vi "Stabilize.vi"() -> ()   [LabVIEW 2013]
uses:
  <vilib>/vision/NI_Vision_Development_Module.lvlib
panel:
  in  "Frame for Template":u32=5000
  out "Match Quality":sgl(graph)
  in  "Stop Updating Panel":bool
  out "Total # Of Frames:":dbl
  out "Stabilized":T1(plugin-control)
  out "Original":T1(plugin-control)
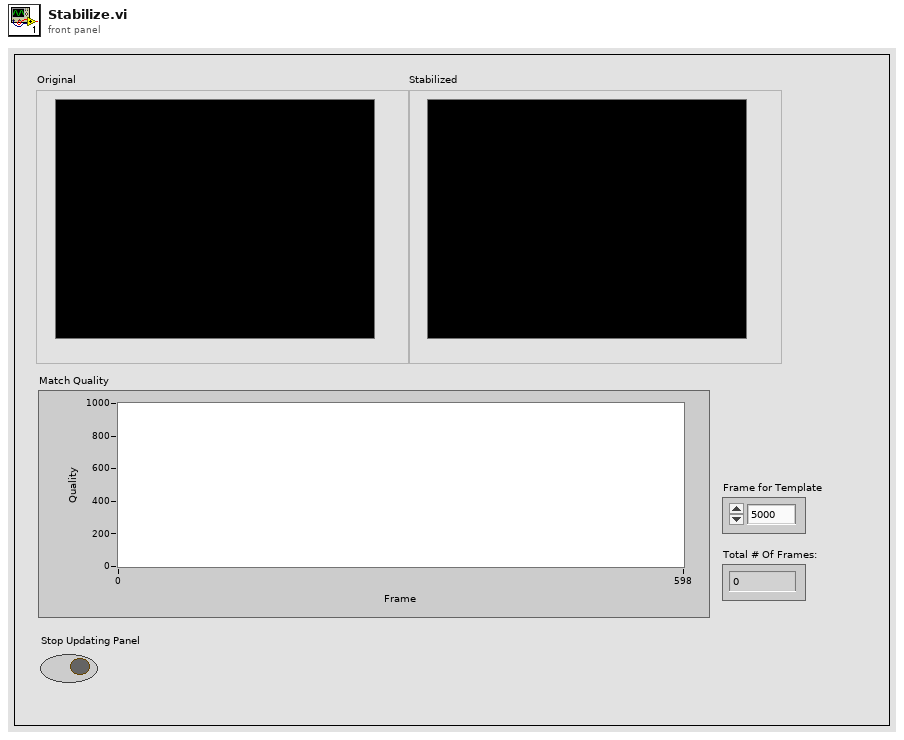
[diagram p1: front panel]
types:
  T1 = typedef "IMAQ Image.ctl" = refnum<image>
  T2 = typedef "AviRefnum.ctl" = refnum<k1>
  T3 = cluster{"width":u32, "height":u32, "framesPerSecond":u32, "compressionFilter":string, "hasData":bool}
  T4 = typedef "IMAQ Rectangle" = cluster{"Left":i32, "Top":i32, "Right":i32, "Bottom":i32, "Rotation":dbl}
  T5 = typedef "ROI Descriptor" = cluster{"Global Rectangle":i32[], "Contours":cluster{"ID":enum32{"External", "Internal"}, "Type":u32, "Coordinates":i32[]}[]}
  T6 = cluster{"Position":cluster{"x":sgl, "y":sgl}, "Angle":sgl, "Scale":sgl, "Score":sgl, "Bounding Box":cluster{"x":sgl, "y":sgl}[]}[]
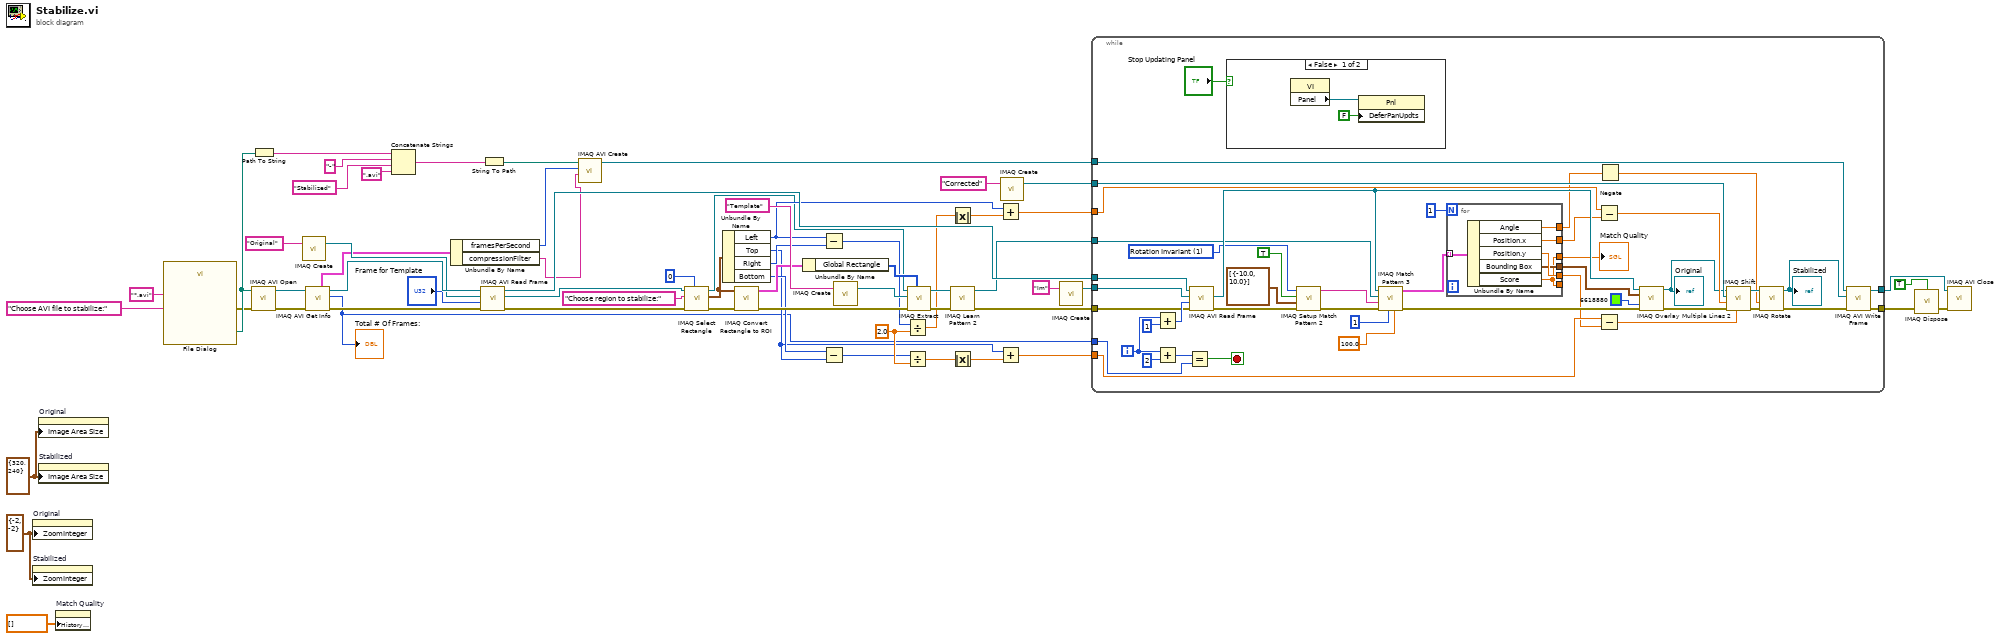
[diagram p0: block diagram]
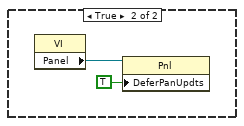
[diagram p2: hidden frame]
diagram:
  w22 = cluster{"X":i32, "Y":i32} {"X"=-2, "Y"=-2} ("ZoomInteger:All Elements")
  w23 = cluster{"Width":u32, "Height":u32} {"Width"=320, "Height"=240} ("Image Area:Size:All Elements")
  w47 = 2.0 ("y")
  n1 = property on="Original" class="ImageControl"("ZoomInteger"=w22) -> ()  [unwired: 2 in, 2 out]
  n2 = property on="Stabilized" class="ImageControl"("ZoomInteger"=w22) -> ()  [unwired: 2 in, 2 out]
  n3 = property on="Original" class="ImageControl"("Image Area Size"=w23) -> ()  [unwired: 2 in, 2 out]
  n4 = property on="Stabilized" class="ImageControl"("Image Area Size"=w23) -> ()  [unwired: 2 in, 2 out]
  n5 = property on="Match Quality" class="WFChart (strict)"("History Data"=sgl[] []) -> ()  [unwired: 2 in, 2 out]
  n6 = call "File Dialog"("prompt"="Choose AVI file to stabilize:", "pattern label"="*.avi") -> ("selected path"=w5:path, "error out"=w3:errorcluster)  [unwired: 10 in, 2 out]
  n7 = call "IMAQ AVI Open"("error in (no error)"=w3, "AVI Path"=w5) -> ("error out"=w62:errorcluster, "Avi Refnum"=w63:T2)  [unwired: 8 in]
  n8 = Path To String(path=w5) -> (string=w10:string)
  n9 = call "IMAQ Create"("Image Name"="Original") -> ("New Image"=w59:T1)  [unwired: 4 in, 1 out]
  n10 = call "IMAQ AVI Get Info"("error in (no error)"=w62, "Avi Refnum"=w63) -> ("error out"=w58:errorcluster, "Number of Frames"=w19:u32, "Avi Refnum (duplicate)"=w61:T2, "Frame Data"=w38:T3)  [unwired: 5 in, 1 out]
  "Total # Of Frames:" <- w19
  n11 = Concatenate Strings(w10, "-" ("string"), "Stabilized" ("string"), ".avi" ("string")) -> (w7:string)
  n12 = Unbundle By Name(w38) -> ("framesPerSecond"=w37:u32, "compressionFilter"=w1:string)
  n13 = call "IMAQ AVI Read Frame"("error in (no error)"=w58, "Frame Number"="Frame for Template", "Image"=w59, "Avi Refnum"=w61) -> ("error out"=w25:errorcluster, "Image Out"=w57:T1, "Avi Refnum (duplicate)"=w48:T2)  [unwired: 4 in, 1 out]
  n14 = String To Path(string=w7) -> (path=w4:path)
  n15 = call "IMAQ AVI Create"("Compression Filter"=w1, "Frames Per Second"=w37, "AVI Path"=w4) -> ("Avi Refnum"=w36:T2)  [unwired: 7 in, 1 out]
  n16 = call "IMAQ Select Rectangle"("Window Number (0...15)"=0, "error in (no error)"=w25, "Prompt"="Choose region to stabilize:", "Image In"=w57) -> ("error out"=w27:errorcluster, "Rectangle"=w18:T4, "Image Out (duplicate)"=w30:T1)  [unwired: 4 in, 1 out]
  n17 = Unbundle By Name(w18) -> ("Left"=w42:i32, "Top"=w41:i32, "Right"=w44:i32, "Bottom"=w43:i32)
  n18 = call "IMAQ Convert Rectangle to ROI"("error in (no error)"=w27, "Rectangle"=w18) -> ("error out"=w53:errorcluster, "ROI Descriptor"=w52:T5)  [unwired: 7 in]
  n19 = Unbundle By Name(w52) -> ("Global Rectangle"=w51:i32[])
  n20 = Subtract(x=w42, y=w44) -> (x-y=w46:i32)
  n21 = Subtract(x=w43, y=w41) -> (x-y=w45:i32)
  n22 = call "IMAQ Create"("Image Name"="Template") -> ("New Image"=w54:T1)  [unwired: 4 in, 1 out]
  n23 = Divide(x=w46, y=w47) -> (x/y=w35:dbl)
  n24 = Divide(x=w45, y=w47) -> (x/y=w33:dbl)
  n25 = call "IMAQ Extract"("Optional Rectangle"=w51, "error in (no error)"=w53, "Image Dst"=w54, "Image Src"=w30) -> ("error out"=w49:errorcluster, "Image Dst Out"=w50:T1)  [unwired: 6 in]
  n26 = Absolute Value(x=w35) -> (abs(x)=w34:dbl)
  n27 = call "IMAQ Learn Pattern 2"("error in (no error)"=w49, "Image"=w50) -> ("error out"=w24:errorcluster, "Template Image Out"=w31:T1)  [unwired: 8 in]
  n28 = Absolute Value(x=w33) -> (abs(x)=w32:dbl)
  n29 = Add(x=w42, y=w34) -> (x+y=w40:dbl)
  n30 = Add(x=w41, y=w32) -> (x+y=w39:dbl)
  n31 = call "IMAQ Create"("Image Name"="Corrected") -> ("New Image"=w14:T1)  [unwired: 4 in, 1 out]
  n32 = call "IMAQ Create"("Image Name"="Im") -> ("New Image"=w16:T1)  [unwired: 4 in, 1 out]
  n33 = while {
    tunnel: w48 -> [w108]
    tunnel: w19 -> [w102]
    tunnel: w31 -> [w87]
    tunnel: w40 -> [w98]
    tunnel: w39 -> [w96]
    tunnel: w36 -> [w94]
    tunnel: w24 -> [w81]
    tunnel: [w84] -> w21
    tunnel: w16 -> [w82]
    tunnel: w14 -> [w79]
    tunnel: [w78] -> w12
    i -> [w105]
    stop <- w101 stop-if-true
    w71 = u16 1 items=["Shift Invariant", "Rotation Invariant"] ("Match Mode")
    n34 = Add(x=w105, y=1) -> (x+y=w106:i32)
    n35 = Add(x=w105, y=2) -> (x+y=w103:i32)
    n36 = Equal?(x=w103, y=w102) -> (x = y?=w101:bool)
    n37 = call "IMAQ AVI Read Frame"("error in (no error)"=w81, "Frame Number"=w106, "Image"=w82, "Avi Refnum"=w108) -> ("error out"=w90:errorcluster, "Image Out"=w92:T1)  [unwired: 4 in, 2 out]
    n38 = case shown="False" "Stop Updating Panel" {
      frame False {
        n39 = property class="VI"() -> ("Panel"=w109:refnum<vi>)  [unwired: 2 in, 2 out]
        n40 = property class="Pnl"(reference=w109, "DeferPanUpdts"=FALSE ("Defer Panel Updates")) -> ()  [unwired: 1 in, 2 out]
      }
      frame True {
        n41 = property class="VI"() -> ("Panel"=w111:refnum<vi>)  [unwired: 2 in, 2 out]
        n42 = property class="Pnl"(reference=w111, "DeferPanUpdts"=TRUE ("Defer Panel Updates")) -> ()  [unwired: 1 in, 2 out]
      }
    }
    n43 = call "IMAQ Setup Match Pattern 2"("error in (no error)"=w90, "Rotation Angle Ranges (degrees)"=cluster{sgl, sgl}[] [{-10.0, 10.0}], "Subpixel Accuracy"=TRUE, "Match Mode"=w71) -> ("error out"=w89:errorcluster, "Match Pattern Setup Data"=w88:string)  [unwired: 6 in]
    n44 = call "IMAQ Match Pattern 3"("Minimum Match Score"=sgl 100.0, "Number of Matches Requested"=1, "error in (no error)"=w89, "Match Pattern Setup Data"=w88, "Template Image"=w87, "Image"=w92) -> ("error out"=w80:errorcluster, "Matches"=w100:T6)  [unwired: 3 in, 1 out]
    n45 = for {
      N: 1 -> [_]
      tunnel: w100 -> [w118] mode=indexing
      tunnel: [w117] -> w77
      tunnel: [w116] -> w76
      tunnel: [w115] -> w93
      tunnel: [w114] -> w85
      tunnel: [w114] -> _
      tunnel: [w113] -> w68
      n46 = Unbundle By Name(w118) -> ("Angle"=w113:sgl, "Position.x"=w117:sgl, "Position.y"=w116:sgl, "Bounding Box"=w115:cluster{"x":sgl, "y":sgl}[], "Score"=w114:sgl)
    }
    "Match Quality" <- w85
    n47 = Subtract(x=w98, y=w77) -> (x-y=w97:dbl)
    n48 = Subtract(x=w96, y=w76) -> (x-y=w95:dbl)
    n49 = Negate(x=w68) -> (-x=w67:sgl)
    n50 = call "IMAQ Overlay Multiple Lines 2"("Image"=w92, "Line End Points"=w93, "Color"=u32 6618880, "error in (no error)"=w80) -> ("Image Out"=w69:T1, "error out"=w70:errorcluster)  [unwired: 10 in]
    "Original" <- w69
    n51 = call "IMAQ Shift"("YOffset"=w95, "error in (no error)"=w70, "XOffset"=w97, "Image Dst"=w79, "Image Src"=w69) -> ("error out"=w74:errorcluster, "Image Dst Out"=w75:T1)  [unwired: 5 in]
    n52 = call "IMAQ Rotate"("error in (no error)"=w74, "Angle (degrees)"=w67, "Image Src"=w75) -> ("error out"=w73:errorcluster, "Image Dst Out"=w72:T1)  [unwired: 7 in]
    "Stabilized" <- w72
    n53 = call "IMAQ AVI Write Frame"("error in (no error)"=w73, "Image"=w72, "Avi Refnum"=w94) -> ("error out"=w78:errorcluster, "Avi Refnum (duplicate)"=w84:T2)  [unwired: 7 in]
  }
  n54 = call "IMAQ Dispose"("All Images? (No)"=TRUE, "error in (no error)"=w12) -> ("error out"=w11:errorcluster)  [unwired: 4 in]
  n55 = call "IMAQ AVI Close"("error in (no error)"=w11, "Avi Refnum"=w21) -> ()  [unwired: 9 in, 1 out]
